vi "Keithley 6517A Reset - Preset.vi"(1 "reset/preset":bool, 2 "error in":T1, 3 "GPIB address":string="27") -> (0 "error out":T1)   [LabVIEW 2013]
doc: "This VI for the Keithley 6517A Electrometer allows the operator to send a \"reset\" or \"preset\" command to the unit. The differences between each of these is explained in full in the instruction manual.\n This VI also disables continuous scans and aborts any scan in progress. This is included in this VI in part because the unit often tries to treat the \"reset\" and \"preset\" commands as triggers if a scan is in progress."
panel:
  # "reset\npreset"
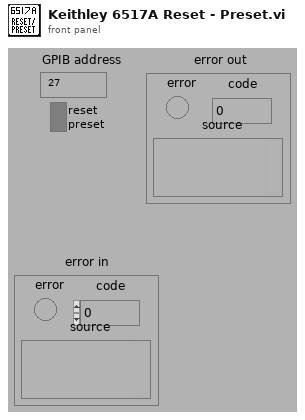
[diagram p1: front panel]
types:
  T1 = cluster{"error":bool, "code":i32, "source":string}
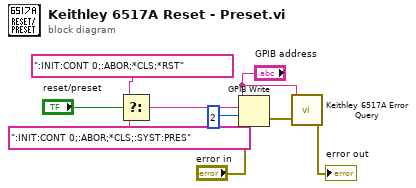
[diagram p0: block diagram]
diagram:
  n1 = Select(t=":INIT:CONT 0;:ABOR;*CLS;*RST", s="reset/preset", f=":INIT:CONT 0;:ABOR;*CLS;:SYST:PRES") -> (s? t:f=w3:string)
  n2 = GPIB Write(0:"GPIB address", 1:w3, 2:2, 3:"error in") -> (6:w6:errorcluster)  [unwired: 1 in, 1 out]
  n3 = call "Keithley 6517A Error Query.vi"("GPIB address"="GPIB address", "error in"=w6) -> ("error out"=→"error out":T1)  [unwired: 1 in, 2 out]
